vi "FPGA_Motor_IO.vi"() -> ()   [LabVIEW 2020]
uses:
  <vilib>/rvi/Emulation/niFpgaGetClockAttributes.vi
  <vilib>/rvi/Emulation/niFpgaSctlEmulationGetInTimedLoop.vi
  <vilib>/rvi/Emulation/niFpgaEmulationReportErrorSimple.vi
  <vilib>/rvi/eio/common/nirviEmuTemplateMethod_errors.vi
  <vilib>/rvi/Emulation/niFpgaCriticalErrorInLSC.vi
  <vilib>/eio/EIONode/EIONode.xnode
panel:
  out "Q":fxp<+/-,24,5>
  out "Pressure":fxp<+/-,24,5>
  out "Encoder1":fxp<+/-,24,5>
  in  "POWER OFF":bool=TRUE
  out "PWM":bool
  in  "Direction":bool
  in  "Enable":bool=TRUE
  in  "duty cycle (periods)":fxp<+,32,0>=0.5 caption="占空比（周期）"
  in  "phase offset (periods)":fxp<+,32,0> caption="相位偏移量（周期）"
  in  "reset":bool caption="重置"
  in  "frequency (periods/tick)":fxp<+,32,0>=2.4999957531690598e-05 caption="频率（周期/滴答）"
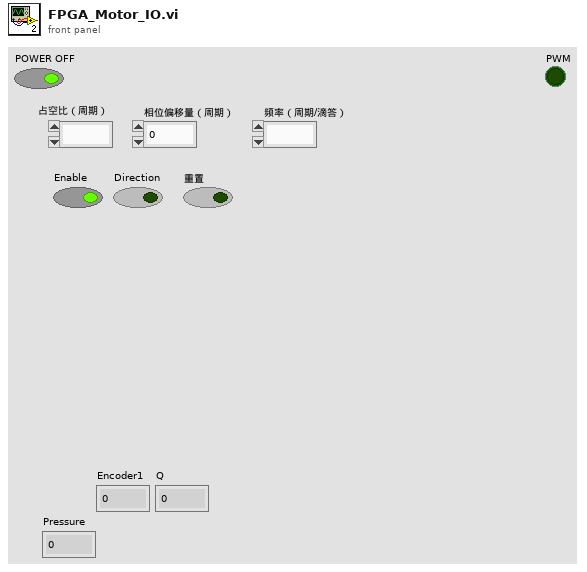
[diagram p1: front panel]
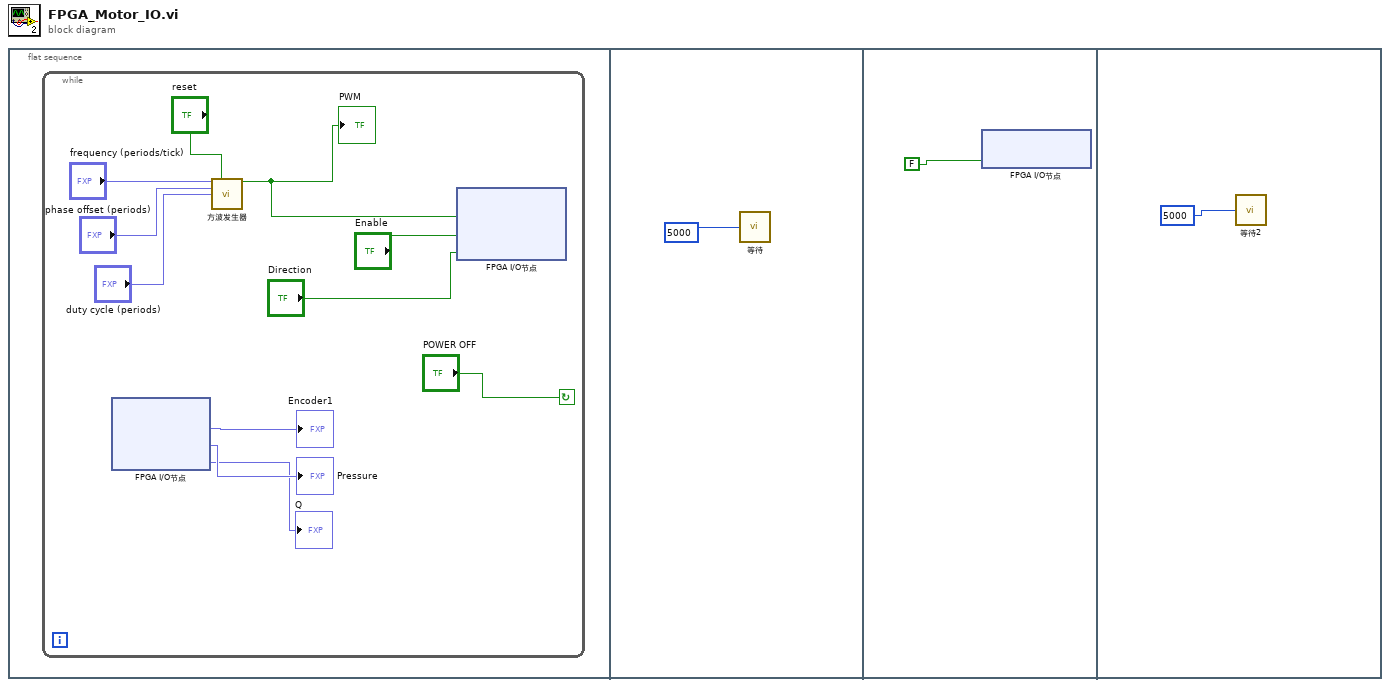
[diagram p0: block diagram]
diagram:
  n1 = flat-sequence {
    frame #0 {
      n2 = while {
        stop <- "POWER OFF" continue-if-true
        n3 = xnode "FPGA I/O节点"() -> ("模块1/AI0"=→"Encoder1":fxp<+/-,24,5>, "模块1/AI1"=→"Pressure":fxp<+/-,24,5>, "模块1/AI2"=→"Q":fxp<+/-,24,5>)  [unwired: 3 in, 3 out]
        n4 = call "方波发生器"("frequency (periods/tick)"="frequency (periods/tick)", "reset"="reset", "phase offset (periods)"="phase offset (periods)", "duty cycle (periods)"="duty cycle (periods)") -> ("square wave out"=w5:bool)  [unwired: 11 in]
        "PWM" <- w5
        n5 = xnode "FPGA I/O节点"("模块6/DIO0"=w5, "模块6/DIO1"="Enable", "模块6/DIO2"="Direction") -> ()  [unwired: 3 in, 3 out]
      }
    }
    frame #1 {
      n6 = call "等待"("Count(uSec)"=i16 5000) -> ()  [unwired: 1 out]
    }
    frame #2 {
      n7 = xnode "FPGA I/O节点"("模块6/DIO1"=FALSE) -> ()  [unwired: 1 in, 1 out]
    }
    frame #3 {
      n8 = call "等待2"("Count(uSec)"=i16 5000) -> ()  [unwired: 1 out]
    }
  }
